vi "ExampleTC01.vi"() -> ()   [LabVIEW 2012]
uses:
  <vilib>/DAQmx/read.llb/DAQmx Read.vi
  <vilib>/DAQmx/read.llb/DAQmx Read (Analog DBL 1Chan 1Samp).vi
  Instance           4 25Saved   LabVIEWTempLogger .vi
  <vilib>/DAQmx/miscellaneous.llb/DAQmx Fill In Error Info.vi
panel:
  in  "physical channel":string="Dev2/ai0"
  in  "thermocouple type":i32(ring)=10072 items=["J"=10072, "K"=10073, "N"=10077, "R"=10082, "S"=10085, "T"=10086, "B"=10047, "E"=10055]
  out "data":dbl format="%0.2f"
  in  "Sampling Interval (s)":dbl=1.0 caption="Delay Time (s)"
  in  "Stop":bool
  # "NI USB-TC01 LabVIEW Temperature Logger"
  # "Switch to the block diagram (Window » Show Block Diagram) to configure the device, thermocouple type, and temperature unit."
  # "© 2010 National Instruments. All rights reserved."
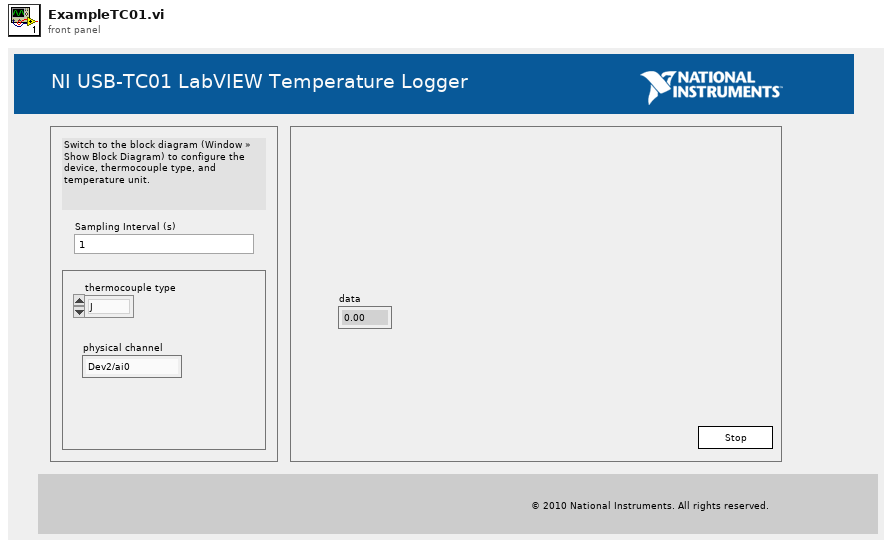
[diagram p1: front panel]
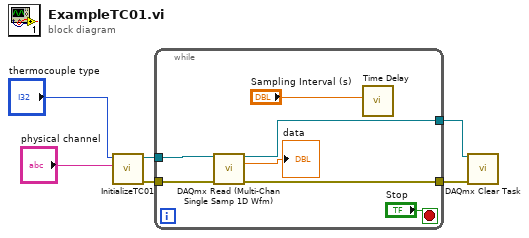
[diagram p0: block diagram]
diagram:
  n1 = call "InitializeTC01.vi"("physical channel"="physical channel", "thermocouple type"="thermocouple type") -> ("error out"=w3:errorcluster, "task out"=w4:refnum<k21>)  [unwired: 8 in]
  n2 = while {
    tunnel: [w10] -> w6
    tunnel: [w9] -> w5
    tunnel: w4 -> [w8]
    tunnel: w3 -> [w7]
    stop <- "Stop" stop-if-true
    n3 = call-poly "DAQmx Read (Multi-Chan Single Samp 1D Wfm).vi"("task/channels in"=w8, "error in"=w7) -> ("task out"=w10:refnum<k21>, "data"=→"data":dbl, "error out"=w9:errorcluster)  [unwired: 11 out]
    n4 = call "Time Delay"("Delay Time (s)"="Sampling Interval (s)") -> ()  [unwired: 10 in, 1 out]
  }
  n5 = call <vilib>:"DAQmx Clear Task.vi"("task in"=w6, "error in"=w5) -> ()  [unwired: 14 out]
